vi "Main.vi"() -> ()   [LabVIEW 2018]
uses:
  controls/sliding_panel_left.ctl
  controls/power_chart.ctl
  controls/max_power_slider.ctl
  controls/tiny_map_icon_basic.ctl
  controls/sliding_panel_right.ctl
  controls/wind_chart.ctl
  controls/sliding_panel_console.ctl
  controls/day_of_month_slider.ctl
  controls/single_multicity_basic.ctl
  controls/plus_basic.ctl
  controls/minus_basic.ctl
  controls/wind_turbine_icon_basic.ctl
  controls/tiny_plots_icon_basic.ctl
  <vilib>/Platform/TimedLoop/XDataNode/timing_clust.ctl
  <vilib>/Platform/TimedLoop/XDataNode/nitl_modes.ctl
  <vilib>/Platform/TimedLoop/XDataNode/wakeup.ctl
  <vilib>/Platform/TimedLoop/XDataNode/XDataNode.xnode
  <vilib>/Platform/TimedLoop/XDataNode/XDNodeRunTimeDep.lvlib
panel:
  in  "show_map":T1
  in  "show_plots":T2
  in  "sliding_panel_console":T3={"Days of Month"=29, "multicity"=FALSE, "plus"=FALSE, "minus"=FALSE} {"Days of Month" min=1 max=30 step=1 scale=0.0..30.0}
  out "sliding_panel_right":T8={"title"="Select a city", "Wind"=[]}
  out "sliding_panel_left":T10={"title"="Power Statistics", "Power"=[], "max_power_slide"=3.1127450980392157, "max_power_digi"=0.13, "max_power_title"="Select a city (# days)"} {"max_power_digi" format="%#_3g"; "max_power_slide" scale=0.0..40.0}
  out "signature":string="Thoric 2011"
  out "title":string="Select a city"
  in  "USA":T13 caption="Texas (USA)"
  in  "costa_rica":T13 caption="Puerto Limon (Costa Rica)"
  in  "brazil":T13 caption="Brasilia (Brazil)"
  in  "south_africa":T13 caption="Cape Good Hope (South Africa)"
  in  "australia":T13 caption="Marrara (Australia)"
  in  "japan":T13 caption="Ise Bay (Japan)"
  in  "india":T13 caption="Mumbai (India)"
  in  "israel":T13 caption="Sde-Dov (Israel)"
  in  "germany":T13 caption="Berlin (Germany)"
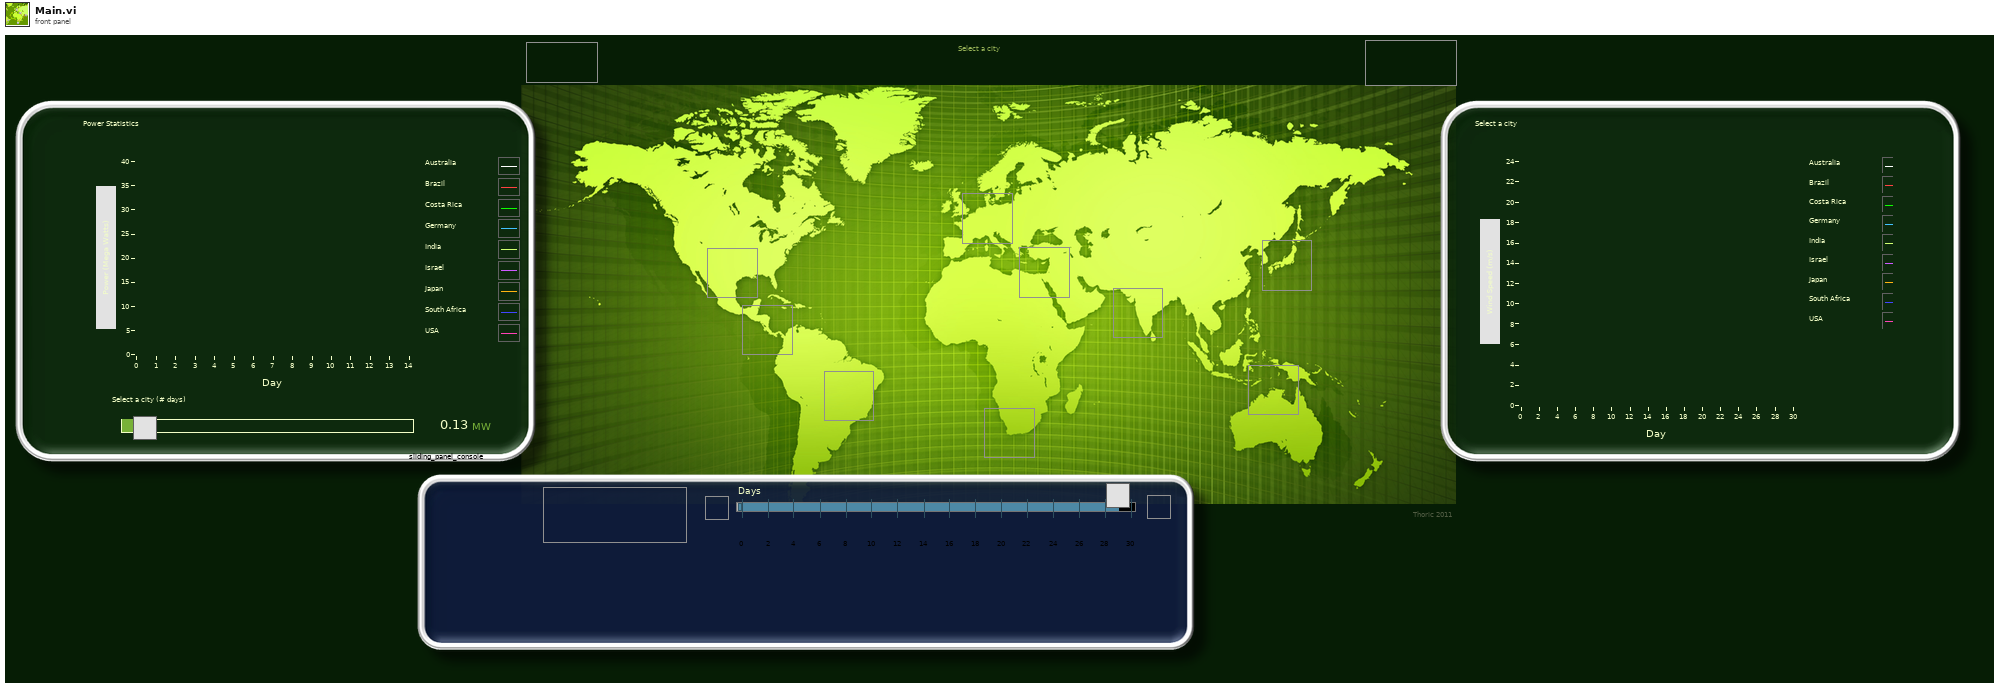
[diagram p1: front panel]
types:
  T1 = typedef "tiny_map_icon_basic.ctl" = bool
  T2 = typedef "tiny_plots_icon_basic.ctl" = bool
  T3 = typedef "sliding_panel_console.ctl" = cluster{"Days of Month":T4, "multicity":T5, "plus":T6, "minus":T7}
  T4 = typedef "day_of_month_slider.ctl" = i32
  T5 = typedef "single_multicity_basic.ctl" = bool
  T6 = typedef "plus_basic.ctl" = bool
  T7 = typedef "minus_basic.ctl" = bool
  T8 = typedef "sliding_panel_right.ctl" = cluster{"title":string, "Wind":T9}
  T9 = typedef "wind_chart.ctl" = dbl[][]
  T10 = typedef "sliding_panel_left.ctl" = cluster{"title":string, "Power":T11, "max_power_slide":T12, "max_power_digi":dbl, "max_power_title":string}
  T11 = typedef "power_chart.ctl" = dbl[][]
  T12 = typedef "max_power_slider.ctl" = dbl
  T13 = typedef "wind_turbine_icon_basic.ctl" = bool
  T14 = enum8{"Enabled", "Disabled", "Disabled and Grayed Out"}
  T15 = typedef "XDNodeRunTimeDep.lvlib/timing_clust.ctl" = cluster{"Expected End [f-1]":u64, "Actual End [f-1]":u64, "Finished Late? [f-1]":bool, "Expected End [i-1]":u64, "Actual End [i-1]":u64, "Finished Late? [i-1]":bool, "Expected Start [i]":u64, "Actual Start [i]":u64, "Expected Start [f]":u64, "Actual Start [f]":u64, "Source Name":string, "Structure Name":string, "Period":i64, "Deadline":i64, "Offset":i64, "Start":i64, "Priority":i32, "Timeout":i32, "Mode":T16, "Wakeup Reason":T17, "Error":errorcluster, "Source Type":string, "Secondary Source Type":string, "Global End Time":u64, "Global Start Time":u64, "Frame Duration":u64, "Iteration Duration":u64, "Assigned CPU":i32, "I/O Scan Engine Mode":u32}
  T16 = typedef "XDNodeRunTimeDep.lvlib/nitl_modes.ctl" = enum32{"No Change", "Process missed periods, maintain original phase", "Discard missed periods, maintain original phase", "Process missed periods, ignore original phase", "Discard missed periods, ignore original phase"}
  T17 = typedef "XDNodeRunTimeDep.lvlib/wakeup.ctl" = enum32{"Normal", "Aborted", "Asynchronous wakeup", "Timing source error", "Timed loop error", "Timeout"}
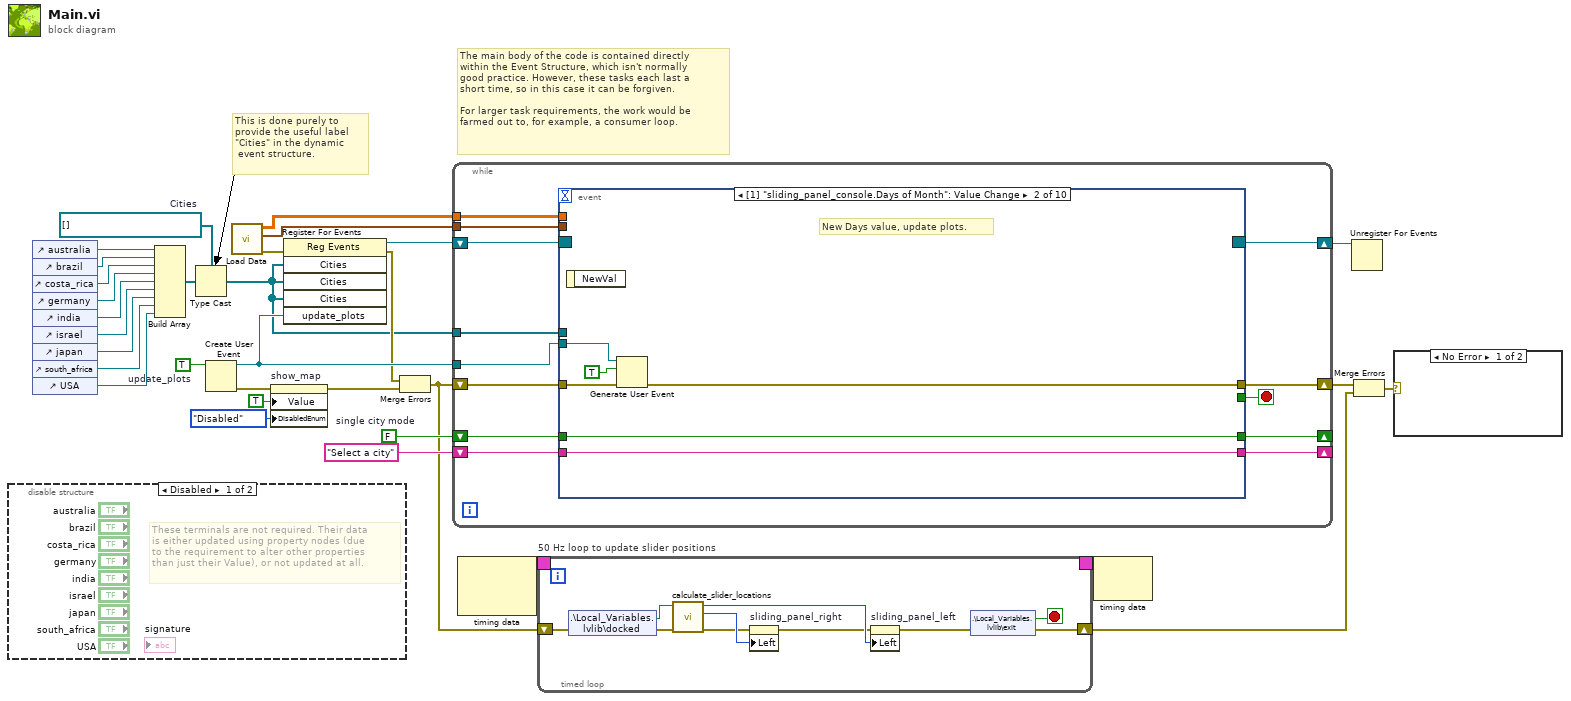
[diagram p0: block diagram]
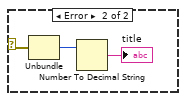
[diagram p3: hidden frame]
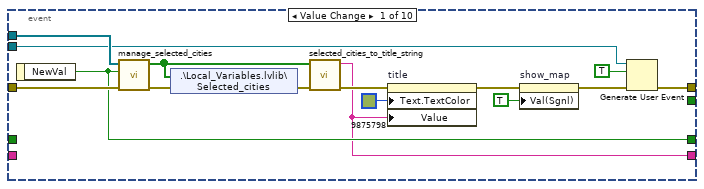
[diagram p4: hidden frame]
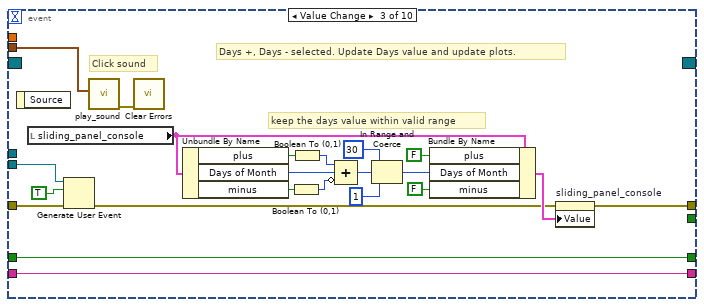
[diagram p5: hidden frame]
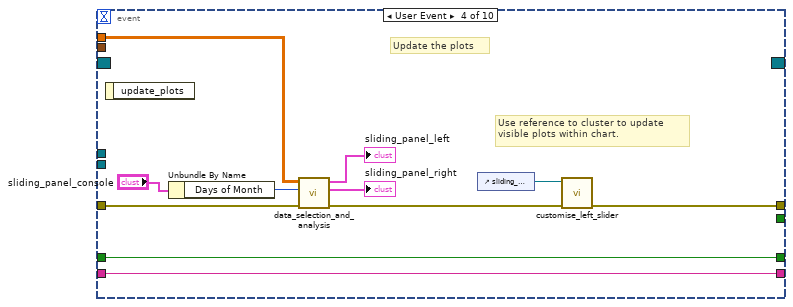
[diagram p6: hidden frame]
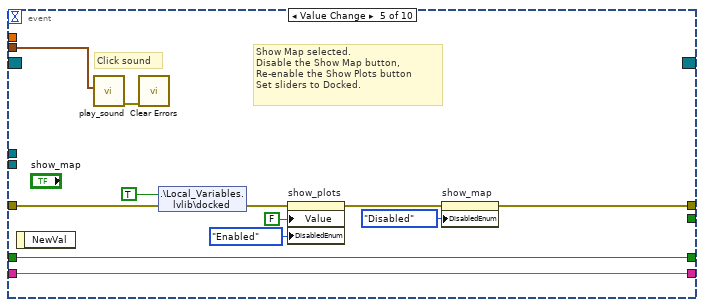
[diagram p7: hidden frame]
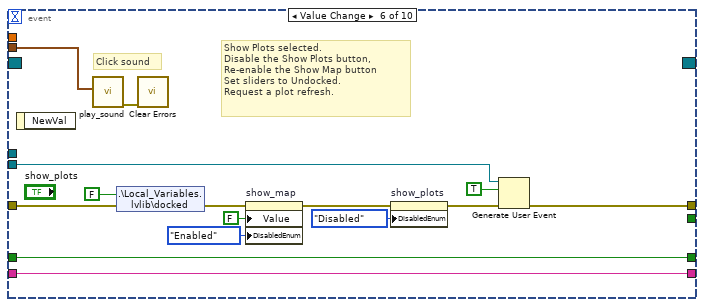
[diagram p8: hidden frame]
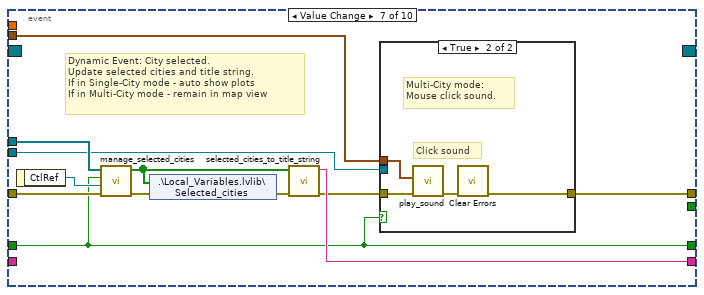
[diagram p9: hidden frame]
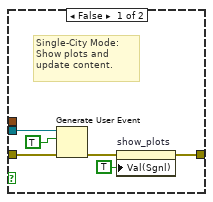
[diagram p10: hidden frame]
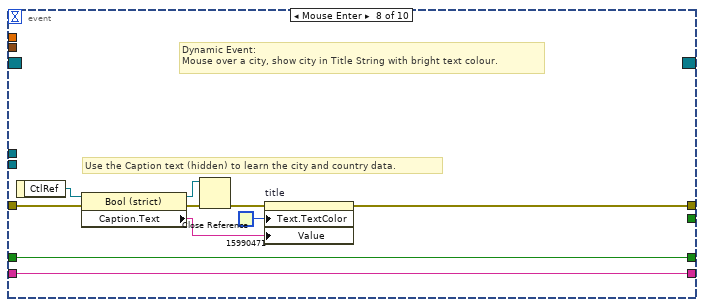
[diagram p11: hidden frame]
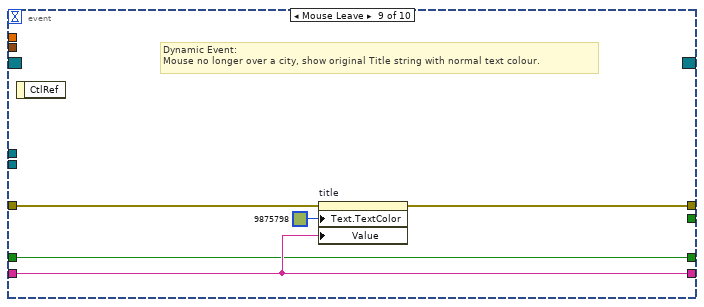
[diagram p12: hidden frame]
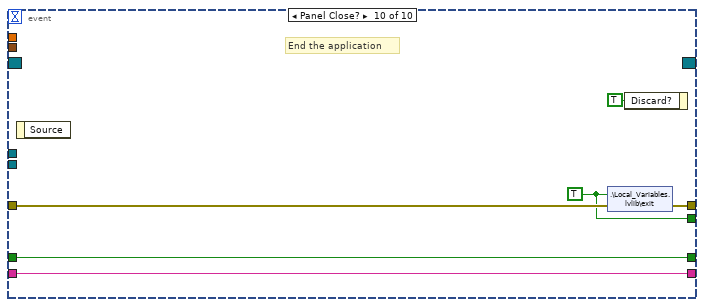
[diagram p13: hidden frame]
diagram:
  w5 = refnum<vi>[] []  # Cities
  w15 = T5 FALSE  # single city mode
  w18 = TRUE  # update_plots
  # "The main body of the code is contained directly\nwithin the Event Structure, which isn't normally\ngood practice. However, these tasks each last a\nshort time, so in this case it can be forgiven.\n\nFor larger task requirements, the work would be\nfarmed out to, for example, a consumer loop."
  # "This is done purely to\nprovide the useful label\n\"Cities\" in the dynamic\n event structure."
  n1 = disable-structure shown="Disabled" {
    frame Disabled {
      # "These terminals are not required. Their data\nis either updated using property nodes (due\nto the requirement to alter other properties\nthan just their Value), or not updated at all."
    }
    frame Enabled {
    }
  }
  n2 = control-ref of="australia"() -> (w29:refnum<vi>)
  n3 = control-ref of="brazil"() -> (w28:refnum<vi>)
  n4 = control-ref of="costa_rica"() -> (w27:refnum<vi>)
  n5 = control-ref of="germany"() -> (w26:refnum<vi>)
  n6 = control-ref of="india"() -> (w25:refnum<vi>)
  n7 = control-ref of="israel"() -> (w24:refnum<vi>)
  n8 = control-ref of="japan"() -> (w23:refnum<vi>)
  n9 = control-ref of="south_africa"() -> (w22:refnum<vi>)
  n10 = control-ref of="USA"() -> (w21:refnum<vi>)
  n11 = Build Array(w29, w28, w27, w26, w25, w24, w23, w22, w21) -> (w7:refnum<vi>[])
  n12 = Type Cast(type=w5, x=w7) -> (*(type *) &x=w6:refnum<vi>[])
  n13 = Create User Event(user event datatype=w18) -> (user event=w17:refnum<user-event>, error out=w2:errorcluster)  [unwired: 1 in]
  n14 = call "Load Data.vi"() -> ("error out"=w13:errorcluster, "Sound WAV data"=w14:waveform(dbl)[], "Wind Data"=w16:dbl[][])  [unwired: 9 in]
  n15 = property on="show_map" class="Bool (strict)"(error in=w2, "Value"=TRUE, "DisabledEnum"=T14."Disabled" ("Disabled")) -> (error out=w1:errorcluster)  [unwired: 1 in, 1 out]
  n16 = register-events(error in=w13, w6, w6, w6, w17) -> (reference out=w30:refnum<event-registration>, error out=w12:errorcluster)  [unwired: 1 in]
  n17 = Merge Errors(w12, w1) -> (w11:errorcluster)
  n18 = while {
    shift-right: [w44] -> w10
    shift-left: w11 -> [w45]
    shift-right: [w41] -> w20
    shift-left: w30 -> [w42]
    shift-right: [w39] -> _
    shift-left: "Select a city" ("title") -> [w40]
    shift-right: [w37] -> _
    shift-left: w15 -> [w38]
    tunnel: w6 -> [w36]
    tunnel: w17 -> [w35]
    tunnel: w16 -> [w34]
    tunnel: w14 -> [w33]
    stop <- w43 stop-if-true
    n19 = event shown="[1] \"sliding_panel_console.Days of Month\": Value Change" {
      selector: w42 -> [_ _ _ _ _ _ _ _ _ _]
      dyn-events: [_ _ _ _ _ _ _ _ _ _] -> w41
      timeout: _ -> [_ _ _ _ _ _ _ _ _ _]
      tunnel: w45 -> [w60 w63 w74 w97 w109 w124 w134 w152 w162 w168]
      tunnel: [w48 w61 w86 w89 w103 w121 w129 w156 w161 w169] -> w44
      tunnel: [_ _ _ _ _ _ _ _ _ w167] -> w43
      tunnel: w40 -> [_ w66 w88 w99 w111 w126 _ w157 w160 w165]
      tunnel: [w52 w66 w88 w99 w111 w126 w137 w157 w160 w165] -> w39
      tunnel: w38 -> [_ w65 w87 w98 w110 w125 w131 w153 w159 w164]
      tunnel: [w59 w65 w87 w98 w110 w125 w131 w153 w159 w164] -> w37
      tunnel: w36 -> [w58 _ _ _ _ _ w136 _ _ _]
      tunnel: w35 -> [w47 w62 w72 _ _ w117 w127 _ _ _]
      tunnel: w34 -> [_ _ _ w96 _ _ _ _ _ _]
      tunnel: w33 -> [_ _ w67 _ w100 w112 w128 _ _ _]
      event Value Change {
        n20 = event-data() -> ("NewVal"=w59:T5)  [unwired: 1 in]
        n21 = call "manage_selected_cities.vi"("error in"=w60, "multicity"=w59, "Selected_cities_refs[]"=w58) -> ("error out"=w57:errorcluster, "Selected_Cities[]"=w55:T13[])  [unwired: 7 in]
        n22 = shared-variable ".\\Local_Variables.lvlib\\Selected_cities"(w55, error in=w57) -> (error out=w56:errorcluster)
        n23 = call "selected_cities_to_title_string.vi"("error in"=w56, "selected_cities"=w55) -> ("error out"=w53:errorcluster, "title_string"=w52:string)  [unwired: 8 in]
        n24 = property on="title" class="Str"(error in=w53, "Text.TextColor"=u32 9875798, "Value"=w52) -> (error out=w51:errorcluster)  [unwired: 1 in, 1 out]
        n25 = property on="show_map" class="Bool (strict)"(error in=w51, "Val(Sgnl)"=TRUE ("docked")) -> (error out=w49:errorcluster)  [unwired: 1 in, 1 out]
        n26 = Generate User Event(user event=w47, event data cluster=TRUE ("event data"), error in=w49) -> (error out=w48:errorcluster)  [unwired: 1 in, 1 out]
      }
      event Value Change {
        # "New Days value, update plots."
        n27 = event-data() -> ()  [unwired: 1 in, 1 out]
        n28 = Generate User Event(user event=w62, event data cluster=TRUE ("event data"), error in=w63) -> (error out=w61:errorcluster)  [unwired: 1 in, 1 out]
      }
      event Value Change {
        # "keep the days value within valid range"
        # "Days +, Days - selected. Update Days value and update plots."
        # "Click sound"
        n29 = event-data() -> ()  [unwired: 1 in, 1 out]
        n30 = local read "sliding_panel_console"() -> (w85:T3)
        n31 = Generate User Event(user event=w72, event data cluster=TRUE ("event data"), error in=w74) -> (error out=w73:errorcluster)  [unwired: 1 in, 1 out]
        n32 = call "play_sound.vi"("Data"=w67) -> ("error out"=w68:errorcluster)  [unwired: 9 in]
        n33 = call <vilib>:"Clear Errors.vi"("error in (no error)"=w68) -> ()  [unwired: 5 in, 2 out]
        n34 = Unbundle By Name(w85) -> ("plus"=w81:T6, "Days of Month"=w82:T4, "minus"=w79:T7)
        n35 = Boolean To (0,1)(Boolean=w79) -> (0, 1=w78:i16)
        n36 = Boolean To (0,1)(Boolean=w81) -> (0, 1=w80:i16)
        n37 = Compound Arithmetic op=ADD(w80, w82, invert w78) -> (w83:T4)
        n38 = In Range and Coerce(upper limit=T4 30, x=w83, lower limit=T4 1) -> (coerced(x)=w71:T4)  [unwired: 1 out]
        n39 = Bundle By Name(cluster=w85, "plus"=T6 FALSE, "Days of Month"=w71, "minus"=T7 FALSE) -> (w84:T3)
        n40 = property on="sliding_panel_console" class="Clust (strict)"(error in=w73, "Value"=w84) -> (error out=w86:errorcluster)  [unwired: 1 in, 1 out]
      }
      event User Event {
        # "Use reference to cluster to update\nvisible plots within chart."
        # "Update the plots"
        n41 = event-data() -> ()  [unwired: 1 in, 1 out]
        n42 = Unbundle By Name("sliding_panel_console") -> ("Days of Month"=w94:T4)
        n43 = call "data_selection_and_analysis.vi"("error in"=w97, "days"=w94, "wind data in"=w96) -> ("error out"=w90:errorcluster, "sliding_panel_right"=→"sliding_panel_right":T8, "left_pane_cluster"=→"sliding_panel_left":T10)  [unwired: 6 in]
        n44 = control-ref of="sliding_panel_left"() -> (w91:refnum<vi>)
        n45 = call "customise_left_slider.vi"("error in"=w90, "slide_left_ref"=w91) -> ("error out"=w89:errorcluster)  [unwired: 9 in]
      }
      event Value Change {
        # "Show Map selected.\nDisable the Show Map button,\nRe-enable the Show Plots button\nSet sliders to Docked."
        # "Click sound"
        n46 = event-data() -> ()  [unwired: 1 in, 1 out]
        n47 = call "play_sound.vi"("Data"=w100) -> ("error out"=w101:errorcluster)  [unwired: 9 in]
        n48 = call <vilib>:"Clear Errors.vi"("error in (no error)"=w101) -> ()  [unwired: 5 in, 2 out]
        n49 = shared-variable ".\\Local_Variables.lvlib\\docked"(TRUE, error in=w109) -> (error out=w107:errorcluster)
        n50 = property on="show_plots" class="Bool (strict)"(error in=w107, "Value"=FALSE ("hide_map"), "DisabledEnum"=T14."Enabled" ("Disabled")) -> (error out=w104:errorcluster)  [unwired: 1 in, 1 out]
        n51 = property on="show_map" class="Bool (strict)"(error in=w104, "DisabledEnum"=T14."Disabled" ("Disabled")) -> (error out=w103:errorcluster)  [unwired: 1 in, 1 out]
      }
      event Value Change {
        # "Show Plots selected.\nDisable the Show Plots button,\nRe-enable the Show Map button\nSet sliders to Undocked.\nRequest a plot refresh."
        # "Click sound"
        n52 = event-data() -> ()  [unwired: 1 in, 1 out]
        n53 = call "play_sound.vi"("Data"=w112) -> ("error out"=w113:errorcluster)  [unwired: 9 in]
        n54 = shared-variable ".\\Local_Variables.lvlib\\docked"(FALSE, error in=w124) -> (error out=w120:errorcluster)
        n55 = call <vilib>:"Clear Errors.vi"("error in (no error)"=w113) -> ()  [unwired: 5 in, 2 out]
        n56 = property on="show_map" class="Bool (strict)"(error in=w120, "Value"=FALSE, "DisabledEnum"=T14."Enabled" ("Disabled")) -> (error out=w116:errorcluster)  [unwired: 1 in, 1 out]
        n57 = property on="show_plots" class="Bool (strict)"(error in=w116, "DisabledEnum"=T14."Disabled" ("Disabled")) -> (error out=w115:errorcluster)  [unwired: 1 in, 1 out]
        n58 = Generate User Event(user event=w117, event data cluster=TRUE ("event data"), error in=w115) -> (error out=w121:errorcluster)  [unwired: 1 in, 1 out]
      }
      event Value Change {
        # "Dynamic Event: City selected.\nUpdate selected cities and title string.\nIf in Single-City mode - auto show plots\nIf in Multi-City mode - remain in map view"
        n59 = event-data() -> ("CtlRef"=w132:refnum<vi>)  [unwired: 1 in]
        n60 = call "manage_selected_cities.vi"("error in"=w134, "selected_city"=w132, "multicity"=w131, "Selected_cities_refs[]"=w136) -> ("error out"=w133:errorcluster, "Selected_Cities[]"=w135:T13[])  [unwired: 6 in]
        n61 = shared-variable ".\\Local_Variables.lvlib\\Selected_cities"(w135, error in=w133) -> (error out=w138:errorcluster)
        n62 = call "selected_cities_to_title_string.vi"("error in"=w138, "selected_cities"=w135) -> ("error out"=w130:errorcluster, "title_string"=w137:string)  [unwired: 8 in]
        n63 = case shown="True" w131 {
          tunnel: w130 -> [w140 w146]
          tunnel: [w143 w145] -> w129
          tunnel: w127 -> [w141 _]
          tunnel: w128 -> [_ w147]
          frame False {
            # "Single-City Mode:\nShow plots and\nupdate content."
            n64 = Generate User Event(user event=w141, event data cluster=TRUE ("event data"), error in=w140) -> (error out=w139:errorcluster)  [unwired: 1 in, 1 out]
            n65 = property on="show_plots" class="Bool (strict)"(error in=w139, "Val(Sgnl)"=TRUE ("docked")) -> (error out=w143:errorcluster)  [unwired: 1 in, 1 out]
          }
          frame True {
            # "Multi-City mode:\nMouse click sound."
            # "Click sound"
            n66 = call "play_sound.vi"("error in"=w146, "Data"=w147) -> ("error out"=w148:errorcluster)  [unwired: 8 in]
            n67 = call <vilib>:"Clear Errors.vi"("error in (no error)"=w148) -> ("error out"=w145:errorcluster)  [unwired: 5 in, 1 out]
          }
        }
      }
      event Mouse Enter {
        # "Use the Caption text (hidden) to learn the city and country data."
        # "Dynamic Event:\nMouse over a city, show city in Title String with bright text colour."
        n68 = event-data() -> ("CtlRef"=w158:refnum<vi>)  [unwired: 1 in]
        n69 = property class="Bool (strict)"(reference=w158, error in=w152) -> (reference out=w150:refnum<vi>, error out=w151:errorcluster, "Caption.Text"=w154:string)
        n70 = Close Reference(reference=w150, error in (no error)=w151) -> (error out=w149:errorcluster)
        n71 = property on="title" class="Str"(error in=w149, "Text.TextColor"=u32 15990471, "Value"=w154) -> (error out=w156:errorcluster)  [unwired: 1 in, 1 out]
      }
      event Mouse Leave {
        # "Dynamic Event:\nMouse no longer over a city, show original Title string with normal text colour."
        n72 = event-data() -> ()  [unwired: 1 in, 1 out]
        n73 = property on="title" class="Str"(error in=w162, "Text.TextColor"=u32 9875798, "Value"=w160) -> (error out=w161:errorcluster)  [unwired: 1 in, 1 out]
      }
      event Panel Close? {
        w167 = TRUE ("exit")
        # "End the application"
        n74 = event-data() -> ()  [unwired: 1 in, 1 out]
        n75 = shared-variable ".\\Local_Variables.lvlib\\exit"(w167, error in=w168) -> (error out=w169:errorcluster)
        n76 = event-data("Discard?"=TRUE) -> ()  [unwired: 1 in, 1 out]
      }
    }
  }
  n77 = node-c288() -> (w32:T15)  [unwired: 2 in]
  n78 = timed-loop "50 Hz loop to update slider positions" {
    timing: w32 -> [_]
    timing-out: [_] -> w31
    shift-right: [w170] -> w9
    shift-left: w11 -> [w171]
    stop <- w176 stop-if-true
    n79 = shared-variable ".\\Local_Variables.lvlib\\docked"(error in=w171) -> (w177:bool, error out=w175:errorcluster)
    n80 = call "calculate_slider_locations.vi"("error in"=w175, "Docked? (F)"=w177) -> ("error out"=w174:errorcluster, "sliding_panel_right_coord"=w178:i32, "sliding_panel_left_coord"=w179:i32)  [unwired: 7 in]
    n81 = property on="sliding_panel_right" class="Clust (strict)"(error in=w174, "Left"=w178) -> (error out=w173:errorcluster)  [unwired: 1 in, 1 out]
    n82 = property on="sliding_panel_left" class="Clust (strict)"(error in=w173, "Left"=w179) -> (error out=w172:errorcluster)  [unwired: 1 in, 1 out]
    n83 = shared-variable ".\\Local_Variables.lvlib\\exit"(error in=w172) -> (w176:bool, error out=w170:errorcluster)
  }
  n84 = node-c288(w31) -> ()  [unwired: 1 out]
  n85 = Unregister For Events(event registration refnum=w20) -> ()  [unwired: 1 in, 1 out]
  n86 = Merge Errors(w10, w9) -> (w8:errorcluster)
  n87 = case shown="No Error" w8 {
    selector: w8 -> [_ w184]
    frame No Error {
    }
    frame Error {
      n88 = Unbundle(w184) -> ("code"=w183:i32)  [unwired: 2 out]
      n89 = Number To Decimal String(number=w183) -> (decimal integer string=→"title":string)  [unwired: 1 in]
    }
  }
